vi "Update Request data.vi"(10 "RequestData":T1) -> (3 "RequestXML":string)   [LabVIEW 2023, in "MES.lvlib"]
uses:
  MES.lvlib
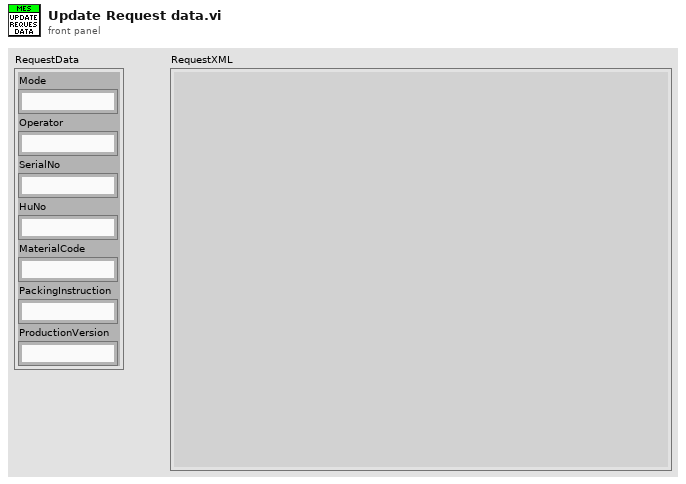
[diagram p1: front panel]
types:
  T1 = cluster{"Mode":string, "Operator":string, "SerialNo":string, "HuNo":string, "MaterialCode":string, "PackingInstruction":string, "ProductionVersion":string}
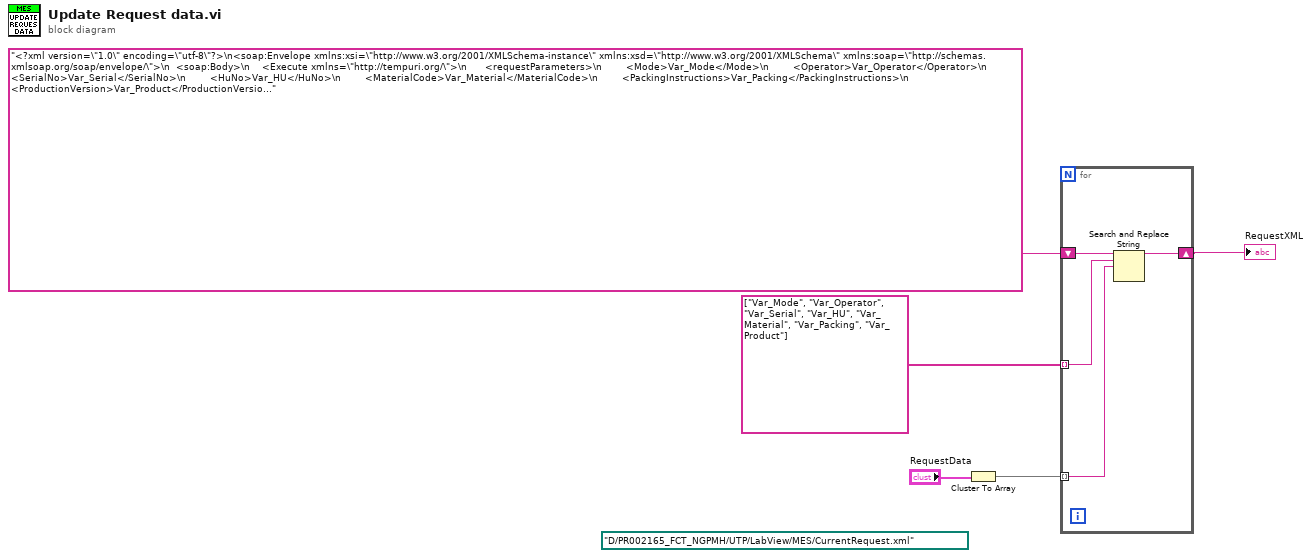
[diagram p0: block diagram]
diagram:
  (unwired) path "D:/PR002165_FCT_NGPMH/UTP/LabView/MES/CurrentRequest.xml" ("file (use dialog)")
  n1 = Cluster To Array(cluster="RequestData") -> (array=w3:string[])
  n2 = for {
    shift-right: [w8] -> w1
    shift-left: "<?xml version=\"1.0\" encoding=\"utf-8\"?>\n<soap:Envelope xmlns:xsi=\"http://www.w3.org/2001/XMLSchema-instance\" xmlns:xsd=\"http://www.w3.org/2001/XMLSchema\" xmlns:soap=\"http://schemas.xmlsoap.org/soap/envelope/\">\n  <soap:Body>\n    <Execute xmlns=\"http://tempuri.org/\">\n      <requestParameters>\n        <Mode>Var_Mode</Mode>\n        <Operator>Var_Operator</Operator>\n        <SerialNo>Var_Serial</SerialNo>\n        <HuNo>Var_HU</HuNo>\n        <MaterialCode>Var_Material</MaterialCode>\n        <PackingInstructions>Var_Packing</PackingInstructions>\n        <ProductionVersion>Var_Product</ProductionVersion>\n      </requestParameters>\n    </Execute>\n  </soap:Body>\n</soap:Envelope>" -> [w9]
    tunnel: w3 -> [w6] mode=indexing
    tunnel: string[] ["Var_Mode", "Var_Operator", "Var_Serial", "Var_HU", "Var_Material", "Var_Packing", "Var_Product"] -> [w7] mode=indexing
    n3 = Search and Replace String(input string=w9, search string=w7, replace string=w6) -> (result string=w8:string)  [unwired: 5 in, 3 out]
  }
  "RequestXML" <- w1
